vi "chart legend delete series.vi"(8 "error in (no error)":errorcluster, 10 "delete_series":i16, 11 "chart":u32) -> (0 "error out":errorcluster, 3 "function return":u32(ring))   [LabVIEW 2015, in "xlsxwriter.lvlib"]
doc: "lxw_error chart_legend_delete_series(lxw_chart chart, int16_t delete_series);"
uses:
  xlsxwriter.lvlib
  xlsxwriter.dll
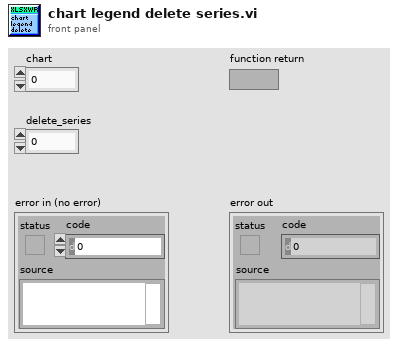
[diagram p1: front panel]
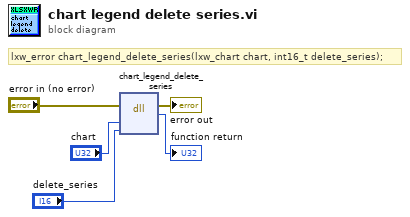
[diagram p0: block diagram]
diagram:
  # "lxw_error chart_legend_delete_series(lxw_chart chart, int16_t delete_series);"
  n1 = dll-call lib="C:/Users/WDAGUtilityAccount/Desktop/lv_vis_added_cell/xlsxwriter.*" fn="chart_legend_delete_series"(error in="error in (no error)", "chart"="chart", "delete_series"="delete_series") -> (error out=→"error out":errorcluster, →"function return":u32)  [unwired: 4 in, 1 out]
